vi "GetMAC.vi"(8 "error in":errorcluster caption="错误输入（无错误）", 10 "PartNum":string="1805", 11 "DevT":string="TBOX") -> (0 "error out":errorcluster caption="错误输出", 3 "MAC":string[](array[string]))   [LabVIEW 2013]
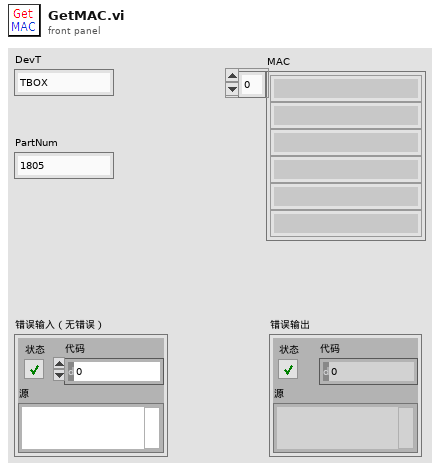
[diagram p1: front panel]
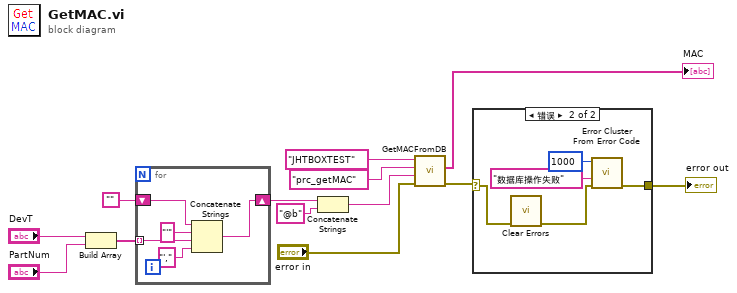
[diagram p0: block diagram]
diagram:
  n1 = Build Array("DevT", "PartNum") -> (w8:string[])
  n2 = for {
    shift-right: [w17] -> w10
    shift-left: "" -> [w18]
    tunnel: w8 -> [w16] mode=indexing
    n3 = Concatenate Strings(w18, "'", w16, "',") -> (w17:string)
  }
  n4 = Concatenate Strings(w10, "@b") -> (w5:string)
  n5 = call "GetMACFromDB.vi"("error in"="error in", "all string"=w5, "Procedure name"="prc_getMAC" ("DSN name"), "DSN name"="JHTBOXTEST") -> ("error out"=w1:errorcluster, "MAC"=→"MAC":string[])  [unwired: 6 in]
  n6 = case shown="错误" w1 {
    selector: w1 -> [w19 w20]
    tunnel: [w19 w24] -> w2
    frame No Error {
    }
    frame Error {
      n7 = call <vilib>:"Clear Errors.vi"("error in (no error)"=w20) -> ("error out"=w21:errorcluster)  [unwired: 6 in]
      n8 = call <vilib>:"Error Cluster From Error Code.vi"("error in (no error)"=w21, "error message (\"\")"="数据库操作失败" ("error message (\"\")"), "error code (0)"=1000) -> ("error out"=w24:errorcluster)  [unwired: 6 in]
    }
  }
  "error out" <- w2
